vi "batch callbyref wait on all.vi"() -> ()   [LabVIEW 2015]
uses:
  result/result.lvclass
  result/result.lvclass/result.ctl
  result/get data.vi
  result/get error.vi
  result/get owning task.vi
  result/get subresults.vi
  standard action/call by reference action/invoke reentrant method in parallel.vi
  task/task.lvclass
  standard reporters/event reporter/event reporter.lvclass
  dispatcher/thread pool.lvclass
  standard action/call by reference action/call function by reference.lvclass
panel:
  out "error":errorcluster
  out "data":variant
  out "Array 2":errorcluster[](array[cluster])
  out "Array":variant[](array[variant])
  out "Time":u32
  out "result":refnum<class "result.lvclass">
  out "error out":errorcluster
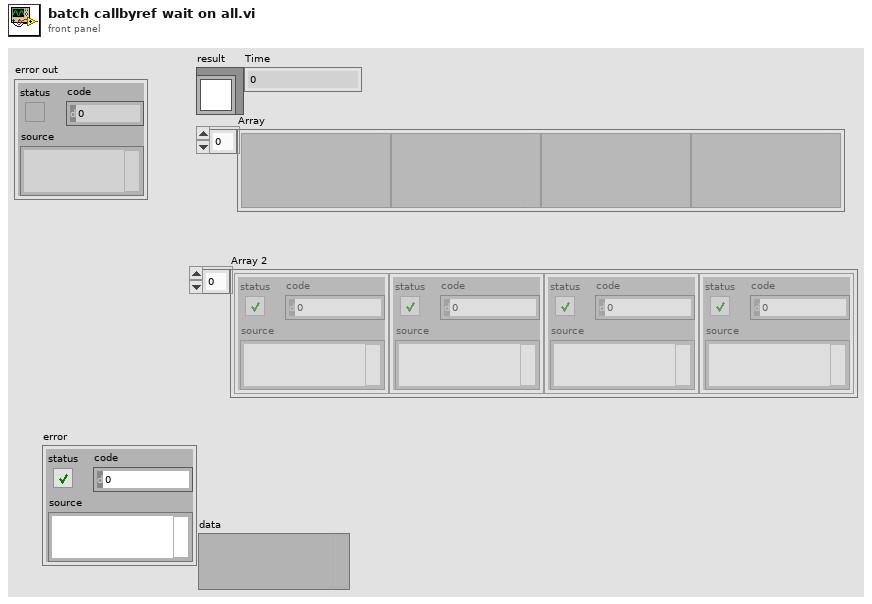
[diagram p1: front panel]
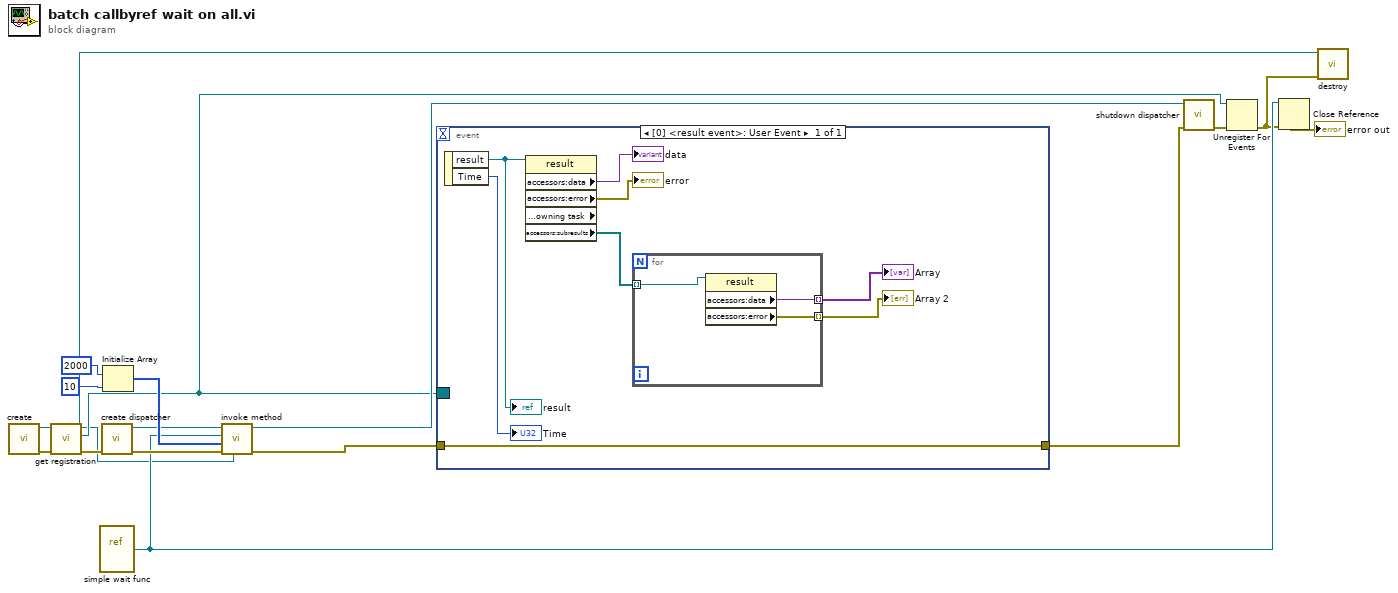
[diagram p0: block diagram]
diagram:
  n1 = call "create.vi"() -> ("error out"=w16:errorcluster, "event reporter out"=w17:refnum<class "event reporter.lvclass">)  [unwired: 10 in]
  n2 = call "get registration.vi"("error in"=w16, "event reporter in"=w17) -> ("error out"=w15:errorcluster, "result registration"=w3:refnum<event-registration>, "event reporter out"=w2:refnum<class "event reporter.lvclass">)  [unwired: 7 in]
  n3 = vi-ref "simple wait func.vi"() -> (w4:refnum<vi>)
  n4 = call "create dispatcher.vi"("error in"=w15) -> ("error out"=w9:errorcluster, "dispatcher"=w6:refnum<class "thread pool.lvclass">)  [unwired: 9 in]
  n5 = Initialize Array(2000, 10 ("dimension size")) -> (w10:i32[])
  n6 = call-poly "invoke method.vi"("results reporter"=w2, "error in"=w9, "parameters"=w10, "VI in"=w4, "thread pool in"=w6) -> ("error out"=w8:errorcluster, "thread pool out"=w7:refnum<class "thread pool.lvclass">)  [unwired: 5 in]
  n7 = event shown="[0] <result event>: User Event" {
    selector: w3 -> [_]
    dyn-events: _ -> [_]
    timeout: _ -> [_]
    tunnel: [w24] -> w13
    tunnel: w8 -> [w24]
    event User Event {
      n8 = event-data() -> ("result"=w23:refnum<class "result.lvclass">, "Time"=→"Time":u32)  [unwired: 1 in]
      "result" <- w23
      n9 = property class="result" props=["accessors:data", "accessors:error", "accessors:owning task", "accessors:subresults"](reference=w23) -> ("accessors:data"=→"data":variant, "accessors:error"=→"error":errorcluster, "accessors:subresults"=w22:refnum<class "result.lvclass">[])  [unwired: 1 in, 3 out]
      n10 = for {
        tunnel: w22 -> [w28] mode=indexing
        tunnel: [w27] -> w21 mode=indexing
        tunnel: [w26] -> w20 mode=indexing
        n11 = property class="result"(reference=w28) -> ("accessors:data"=w27:variant, "accessors:error"=w26:errorcluster)  [unwired: 1 in, 2 out]
      }
      "Array" <- w21
      "Array 2" <- w20
    }
  }
  n12 = call "shutdown dispatcher.vi"("error in"=w13, "thread pool"=w7) -> ("error out"=w14:errorcluster)  [unwired: 9 in]
  n13 = Unregister For Events(event registration refnum=w3, error in=w14) -> (error out=w1:errorcluster)
  n14 = Close Reference(reference=w4, error in (no error)=w1) -> (error out=→"error out":errorcluster)
  n15 = call-dynamic "destroy.vi"("error in"=w1, "event reporter in"=w2) -> ()  [unwired: 9 in, 1 out]
